vi "Get Channels from Line.vi"(11 "Line":T1) -> (3 "Channels":refnum<class "TBM channel.lvclass">[](array[class]))   [LabVIEW 2018, in "Benchmark PID configuration.lvclass"]
doc: "Returns an array of channels for a single line."
uses:
  Benchmark PID configuration.lvclass
  <vilib>/NI/Tag Bus Module Framework/channel/TBM channel.lvclass
  Line.ctl
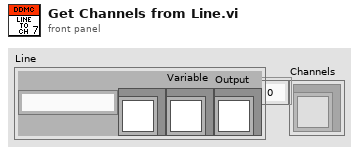
[diagram p1: front panel]
types:
  T1 = typedef "Benchmark PID configuration.lvclass/Line.ctl" = cluster{"PID Name":string, "Setpoint":refnum<class "TBM channel.lvclass">, "Variable":refnum<class "TBM channel.lvclass">, "Output":refnum<class "TBM channel.lvclass">}
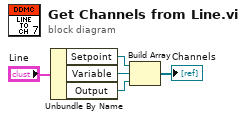
[diagram p0: block diagram]
diagram:
  n1 = Unbundle By Name("Line") -> ("Setpoint"=w3:refnum<class "TBM channel.lvclass">, "Variable"=w2:refnum<class "TBM channel.lvclass">, "Output"=w1:refnum<class "TBM channel.lvclass">)
  n2 = Build Array(w3, w2, w1) -> (→"Channels":refnum<class "TBM channel.lvclass">[])
